vi "Input File Step Iterator.vi"(6 "error in (no error)":errorcluster, 8 "LBCB Input Files":path[](array[path]), 9 "Input File Step Actions":T4) -> (0 "error out":errorcluster, 1 "End of Input File":bool, 2 "Last Step":i32, 3 "Next Step":T1)   [LabVIEW 2009]
uses:
  Input File Step Actions.ctl
  Load Step.ctl
  Target.ctl
  Data Access Objects/Metadata/LBCB Number.ctl
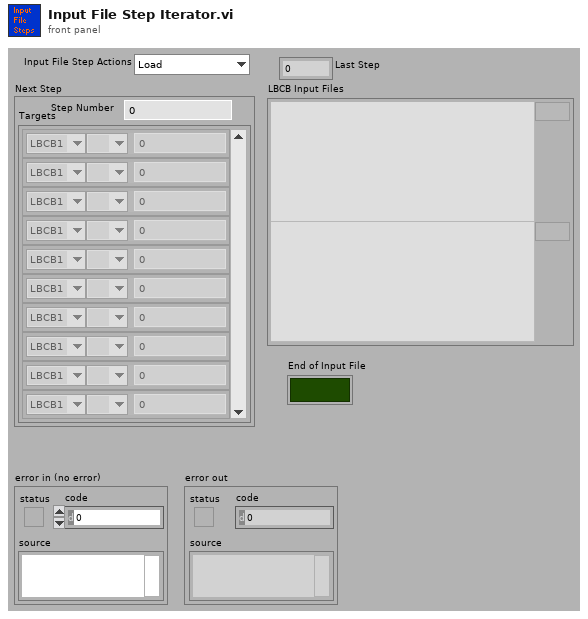
[diagram p1: front panel]
types:
  T1 = typedef "Load Step.ctl" = cluster{"Step Number":u32, "Targets":T2[]}
  T2 = typedef "Target.ctl" = cluster{"LBCB Number":T3, "DOF Vectors":enum16{" ", "Dx", "Dy", "Dz", "Rx", "Ry", "Rz", "Fx", "Fy", "Fz", "Mx", "My", "Mz"}, "Amount":dbl}
  T3 = typedef "LBCB Number.ctl" = enum16{"LBCB1", "LBCB2"}
  T4 = typedef "Input File Step Actions.ctl" = enum16{"Load", "Next Step", "Reset", "Get Step"}
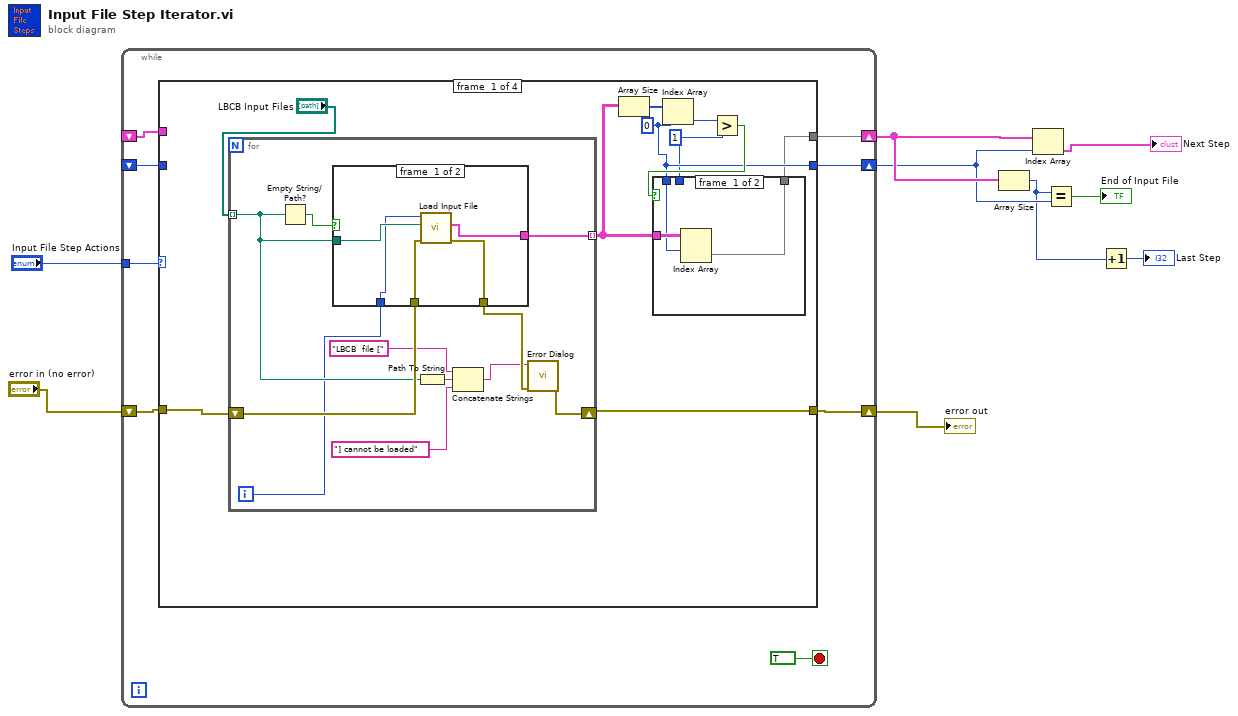
[diagram p0: block diagram]
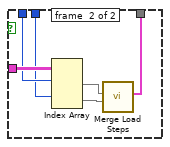
[diagram p2: hidden frame]
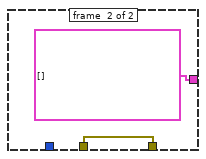
[diagram p3: hidden frame]
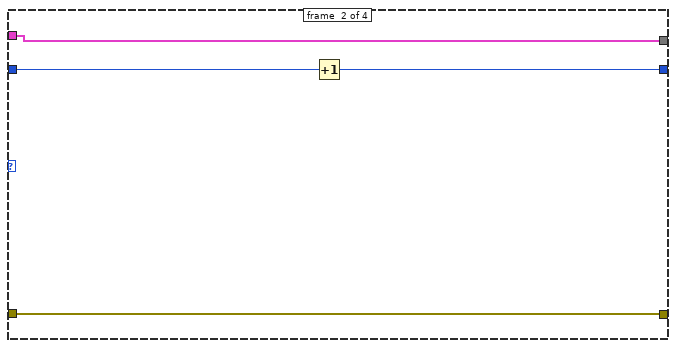
[diagram p4: hidden frame]
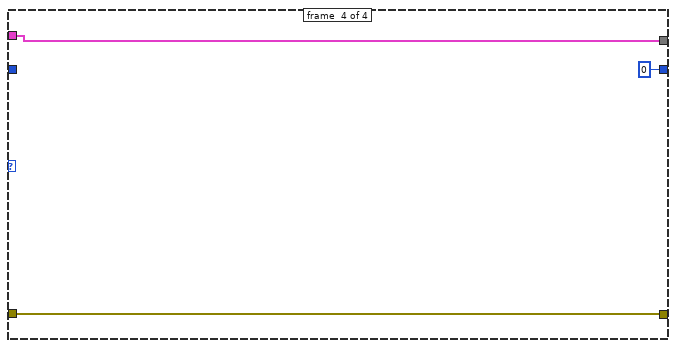
[diagram p6: hidden frame]
diagram:
  n1 = while {
    tunnel: "Input File Step Actions" -> [w16]
    shift-right: [w14] -> w7
    shift-left: "error in (no error)" -> [w15]
    shift-right: [w13] -> w6
    shift-left: _ -> [w11]
    shift-right: [w12] -> w5
    shift-left: _ -> [w10]
    stop <- TRUE stop-if-true
    n2 = case shown="\"Get Step\"" w16 {
      tunnel: w15 -> [w27 w57 w61 w63]
      tunnel: [w25 w57 w61 w63] -> w14
      tunnel: [w18 w55 w60 w64] -> w13
      tunnel: [w20 w56 w59 0] -> w12
      tunnel: w11 -> [_ w55 w60 w64]
      tunnel: w10 -> [_ w58 w59 _]
      frame #0 {
        w19 = 1 ("y")
        w20 = 0 ("index")
        n3 = for {
          tunnel: "LBCB Input Files" -> [w40] mode=indexing
          shift-right: [w39] -> w25
          shift-left: w27 -> [w46]
          tunnel: [w38] -> w21 mode=indexing
          i -> [w37]
          n4 = Empty String/Path?(string/path=w40) -> (empty?=w47:bool)
          n5 = case shown="False" w47 {
            tunnel: w46 -> [w52 w54]
            tunnel: [w51 w54] -> w44
            tunnel: [w50 T1[] [] ("Load Steps")] -> w38
            tunnel: w40 -> [w49 _]
            tunnel: w37 -> [w48 _]
            frame #0 {
              n6 = call "Load Input File.vi"("error in (no error)"=w52, "Path"=w49, "LBCB Filter"=w48) -> ("error out"=w51:errorcluster, "Load Steps"=w50:T1[])  [unwired: 7 out]
            }
            frame #1 {
            }
          }
          n7 = Path To String(path=w40) -> (string=w45:string)
          n8 = Concatenate Strings("LBCB  file [" ("string"), w45, "] cannot be loaded" ("string")) -> (w43:string)
          n9 = call "Error Dialog.vi"("error in (no error)"=w44, "Message"=w43) -> ("error out"=w39:errorcluster)  [unwired: 9 out]
        }
        n10 = Array Size(array=w21) -> (size(s)=w24:i32[])
        n11 = Index Array(array=w24, index=w20) -> (element=w23:i32)
        n12 = Greater?(x=w23, y=w19) -> (0:w22:bool)
        n13 = case shown="False" w22 {
          tunnel: w21 -> [w30 w36]
          tunnel: w20 -> [w29 w35]
          tunnel: w19 -> [_ w34]
          tunnel: [w28 w31] -> w18
          frame #0 {
            n14 = Index Array(array=w30, index (row)=w29) -> (element=w28:T1[])  [unwired: 1 in]
          }
          frame #1 {
            n15 = Index Array(array=w36, index (row) #1=w35, index (row) #2=w34) -> (element #1=w33:T1[], element #2=w32:T1[])  [unwired: 2 in]
            n16 = call "Merge Load Steps.vi"("Load Steps  In 2"=w32, "Load Steps In"=w33) -> ("Load Steps Out"=w31:T1[])  [unwired: 9 out]
          }
        }
      }
      frame #1 {
        n17 = Increment(x=w58) -> (x+1=w56:i32)
      }
      frame #2 {
      }
      frame #3 {
      }
    }
  }
  "error out" <- w7
  n18 = Array Size(array=w6) -> (size(s)=w3:i32)
  n19 = Index Array(array=w6, index=w5) -> (element=→"Next Step":T1)
  n20 = Equal?(x=w3, y=w5) -> (x = y?=→"End of Input File":bool)
  n21 = Increment(x=w3) -> (x+1=→"Last Step":i32)
